vi "KeyboardInput2.vi"(0 "error in (no error)":errorcluster, 1 "Speed step":dbl, 2 "device ID":refnum<k1>) -> (3 "Control cluster":T1 {"Roll" scale=-1.0..1.0; "Pitch" scale=-1.0..1.0; "Vertical Speed" scale=-1.0..1.0; "Yaw Speed" scale=-1.0..1.0}, 4 "error out":errorcluster)   [LabVIEW 2014]
uses:
  <vilib>/Utility/inputDevices.llb/keyboardAcquire.vi
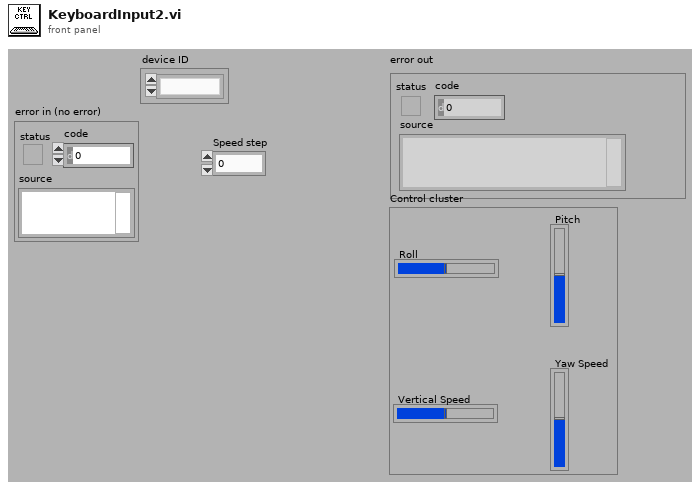
[diagram p1: front panel]
types:
  T1 = cluster{"Roll":dbl, "Pitch":dbl, "Vertical Speed":dbl, "Yaw Speed":dbl}
  T2 = enum16{"0", "1", "2", "3", "4", "5", "6", "7", "8", "9", "A", "B", "C", "D", "E", "F", "G", "H", "I", "J", "K", "L", "M", "N", "O", "P", "Q", "R", "S", "T", "U", "V", "W", "X", "Y", "Z", "F1", "F2", "F3", "F4", "F5", "F6", "F7", "F8", "F9", "F10", "F11", "F12", "F13", "F14", "F15", "ADD", "BACK", "BACKSLASH", "CAPITAL", "COMMA", "DECIMAL", "DELETE", "DIVIDE", "DOWN", "END", "EQUALS", "ESCAPE", "GRAVE (`)", "HOME", "INSERT", "LBRACKET", "LCONTROL", "LEFT", "L ALT", "LSHIFT", "LWIN", "MINUS", "MULTIPLY", "NEXT", "NUMLOCK", "NUMPAD_0", "NUMPAD_1", "NUMPAD_2", "NUMPAD_3", "NUMPAD_4", "NUMPAD_5", "NUMPAD_6", "NUMPAD_7", "NUMPAD_8", "NUMPAD_9", "PAUSE", "PERIOD", "PRIOR (PG UP)", "RBRACKET", "RCONTROL", "RETURN", "RIGHT", "R ALT", "RSHIFT", "RWIN", "SCROLL", "SEMICOLON", "SLASH", "SPACE", "SUBTRACT", "TAB", "UP", "ENTER (num pad)", "' (quote)"}[]
  T3 = enum16{"0", "1", "2", "3", "4", "5", "6", "7", "8", "9", "A", "B", "C", "D", "E", "F", "G", "H", "I", "J", "K", "L", "M", "N", "O", "P", "Q", "R", "S", "T", "U", "V", "W", "X", "Y", "Z", "F1", "F2", "F3", "F4", "F5", "F6", "F7", "F8", "F9", "F10", "F11", "F12", "F13", "F14", "F15", "ADD", "BACK", "BACKSLASH", "CAPITAL", "COMMA", "DECIMAL", "DELETE", "DIVIDE", "DOWN", "END", "EQUALS", "ESCAPE", "GRAVE (`)", "HOME", "INSERT", "LBRACKET", "LCONTROL", "LEFT", "L ALT", "LSHIFT", "LWIN", "MINUS", "MULTIPLY", "NEXT", "NUMLOCK", "NUMPAD_0", "NUMPAD_1", "NUMPAD_2", "NUMPAD_3", "NUMPAD_4", "NUMPAD_5", "NUMPAD_6", "NUMPAD_7", "NUMPAD_8", "NUMPAD_9", "PAUSE", "PERIOD", "PRIOR (PG UP)", "RBRACKET", "RCONTROL", "RETURN", "RIGHT", "R ALT", "RSHIFT", "RWIN", "SCROLL", "SEMICOLON", "SLASH", "SPACE", "SUBTRACT", "TAB", "UP", "ENTER (num pad)", "' (quote)"}
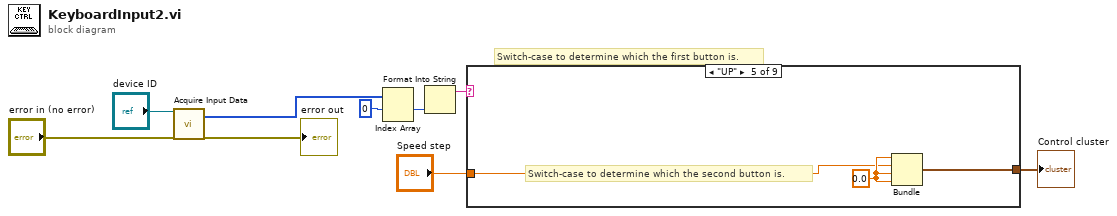
[diagram p0: block diagram]
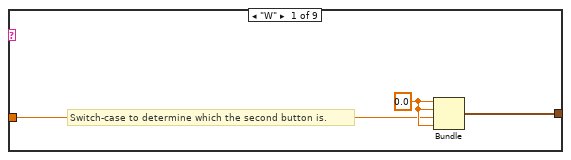
[diagram p2: hidden frame]
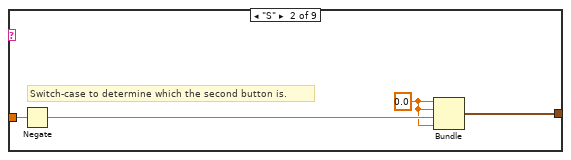
[diagram p3: hidden frame]
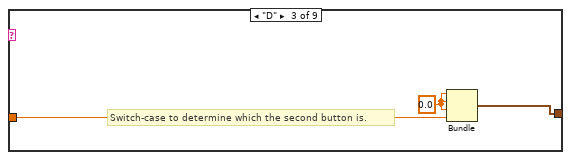
[diagram p4: hidden frame]
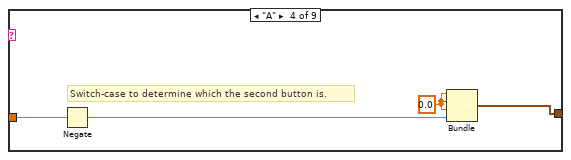
[diagram p5: hidden frame]
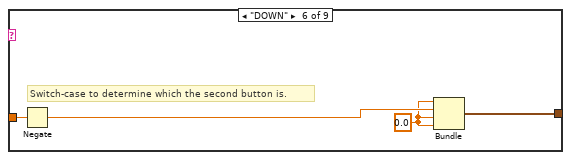
[diagram p6: hidden frame]
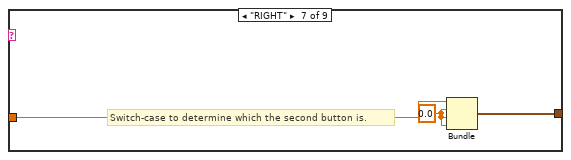
[diagram p7: hidden frame]
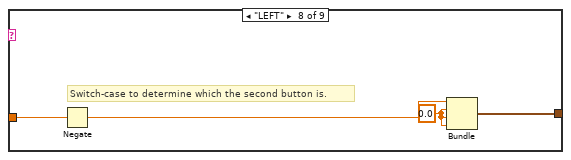
[diagram p8: hidden frame]
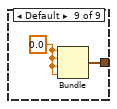
[diagram p9: hidden frame]
diagram:
  # "Switch-case to determine which the first button is."
  n1 = call-poly <vilib>:"Acquire Input Data.vi"("device ID"="device ID", "error in (no error)"="error in (no error)") -> ("keys pressed"=w3:T2, "error out"=→"error out":errorcluster)  [unwired: 15 in, 1 out]
  n2 = Index Array(array=w3, index #1=0) -> (element #1=w7:T3)  [unwired: 1 in, 1 out]
  n3 = Format Into String(w7) -> (resulting string=w9:string)  [unwired: 3 in, 1 out]
  n4 = case shown="\"UP\"" w9 {
    tunnel: [w10 w13 w17 w20 w25 w27 w31 w34 w38] -> w2
    tunnel: "Speed step" -> [w11 w14 w18 w21 w24 w28 w32 w35 _]
    frame "W" {
      w12 = 0.0
      # "Switch-case to determine which the second button is."
      n5 = Bundle(w12, w12, "Speed step"=w11, w12) -> (w10:cluster{dbl, dbl, "Speed step":dbl, dbl})  [unwired: 1 in]
    }
    frame "S" {
      w15 = 0.0
      # "Switch-case to determine which the second button is."
      n6 = Negate(x=w14) -> (-x=w16:dbl)
      n7 = Bundle(w15, w15, w16, w15) -> (w13:cluster{dbl, dbl, dbl, dbl})  [unwired: 1 in]
    }
    frame "D" {
      w19 = 0.0
      # "Switch-case to determine which the second button is."
      n8 = Bundle(w19, w19, w19, "Speed step"=w18) -> (w17:cluster{dbl, dbl, dbl, "Speed step":dbl})  [unwired: 1 in]
    }
    frame "A" {
      w23 = 0.0
      # "Switch-case to determine which the second button is."
      n9 = Negate(x=w21) -> (-x=w22:dbl)
      n10 = Bundle(w23, w23, w23, w22) -> (w20:cluster{dbl, dbl, dbl, dbl})  [unwired: 1 in]
    }
    frame "UP" {
      w26 = 0.0
      # "Switch-case to determine which the second button is."
      n11 = Bundle(w26, "Speed step"=w24, w26, w26) -> (w25:cluster{dbl, "Speed step":dbl, dbl, dbl})  [unwired: 1 in]
    }
    frame "DOWN" {
      w29 = 0.0
      # "Switch-case to determine which the second button is."
      n12 = Negate(x=w28) -> (-x=w30:dbl)
      n13 = Bundle(w29, w30, w29, w29) -> (w27:cluster{dbl, dbl, dbl, dbl})  [unwired: 1 in]
    }
    frame "RIGHT" {
      w33 = 0.0
      # "Switch-case to determine which the second button is."
      n14 = Bundle("Speed step"=w32, w33, w33, w33) -> (w31:cluster{"Speed step":dbl, dbl, dbl, dbl})  [unwired: 1 in]
    }
    frame "LEFT" {
      w36 = 0.0
      # "Switch-case to determine which the second button is."
      n15 = Negate(x=w35) -> (-x=w37:dbl)
      n16 = Bundle(w37, w36, w36, w36) -> (w34:cluster{dbl, dbl, dbl, dbl})  [unwired: 1 in]
    }
    frame Default {
      w39 = 0.0
      n17 = Bundle(w39, w39, w39, w39) -> (w38:cluster{dbl, dbl, dbl, dbl})  [unwired: 1 in]
    }
  }
  "Control cluster" <- w2
